vi "Close Report File.vi"(8 "error in (no error)":errorcluster, 11 "Text Report In":refnum<class "Text Report.lvclass">) -> (0 "error out":errorcluster)   [LabVIEW 2020, in "Reports.lvlib" / "Text Report.lvclass"]
uses:
  Text Report.lvclass
  Text Report.lvclass/Text Report.ctl
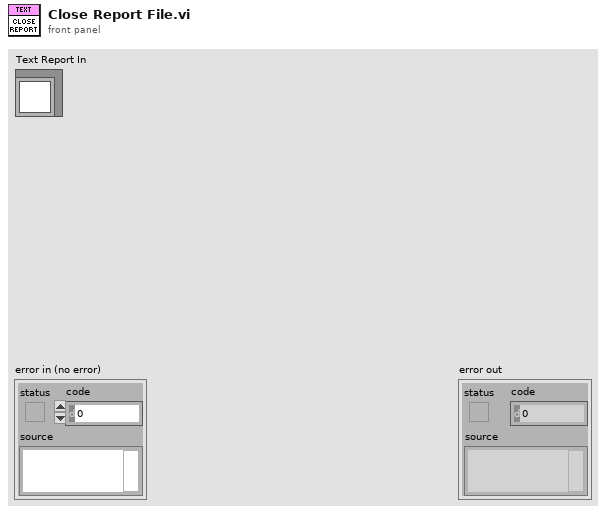
[diagram p1: front panel]
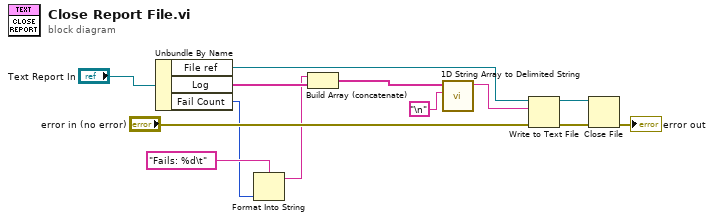
[diagram p0: block diagram]
diagram:
  n1 = Unbundle By Name("Text Report In") -> ("File ref"=w9:refnum<file>, "Log"=w6:string[], "Fail Count"=w1:i32)
  n2 = Format Into String(format string="Fails: %d\t", w1) -> (resulting string=w2:string)  [unwired: 2 in, 1 out]
  n3 = Build Array (concatenate)(w2, w6) -> (w3:string[])
  n4 = call <vilib>:"1D String Array to Delimited String.vi"("delimiter"="\n", "string array"=w3) -> ("delimited string"=w5:string)  [unwired: 9 in]
  n5 = Write to Text File(file (use dialog)=w9, text=w5, error in="error in (no error)") -> (refnum out=w8:refnum<file>, error out=w10:errorcluster)  [unwired: 1 in, 1 out]
  n6 = Close File(refnum=w8, error in=w10) -> (error out=→"error out":errorcluster)  [unwired: 1 out]
